vi "CD Calculations.vi"(10 "AC":dbl, 11 "DC":dbl) -> (3 "CD":dbl)   [LabVIEW 2017, in "Lockin and Keithley Multimeter.lvclass"]
uses:
  Lockin and Keithley Multimeter.lvclass
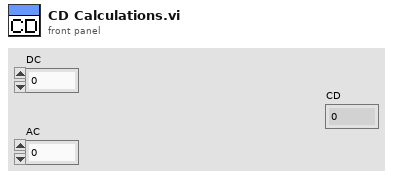
[diagram p1: front panel]
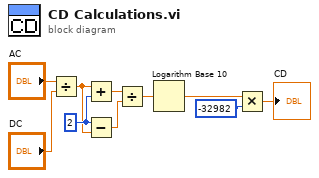
[diagram p0: block diagram]
diagram:
  w6 = 2
  n1 = Divide(x="AC", y="DC") -> (x/y=w5:dbl)
  n2 = Add(x=w5, y=w6) -> (x+y=w8:dbl)
  n3 = Subtract(x=w6, y=w5) -> (x-y=w7:dbl)
  n4 = Divide(x=w8, y=w7) -> (x/y=w4:dbl)
  n5 = Logarithm Base 10(1:w4) -> (0:w3:dbl)
  n6 = Multiply(x=w3, y=-32982) -> (x*y=→"CD":dbl)
